vi "Master on Desktop — копия (2).vi"() -> ()   [LabVIEW 2021]
doc: "Demonstrates how to use Modbus functions to create a master communicating with a Modbus slave. It shows an interactive UI to allow users manually read and write the coils on the slave using TCP connection. Users can also change the timeout for reading operation if the network state is not good."
uses:
  subvis/Modbus API/Modbus API.lvclass/Modbus API.ctl
  subvis/Transmission Data Unit (ADU)/Transmission Data Unit/Transmission Data Unit.lvclass/Transmission Data Unit.ctl
  master/Data Access/Read Timeout/Set Read Timeout.vi
  subvis/Modbus API/Read Transmission Data Unit.vi
  subvis/Modbus API/Write Transmission Data Unit.vi
  subvis/Transmission Data Unit (ADU)/Transmission Data Unit/Data Access/timeouts/Write read operation timeout.vi
  master/Modbus Master.lvclass
  D:/my_projects/projects/Algorithms/Labview/21/Modbus_v2/subvis/Modbus API/Modbus API.lvclass
  master/Create Master Instance (TCP).vi
  subvis/Transmission Data Unit (ADU)/Transmission Data Unit/Transmission Data Unit.lvclass
panel:
  out "timer":u32(graph)
  in  "register values 2":u16[](array[numeric])
  out "register values":u16[](array[numeric])
  in  "Set Read Timeout":bool
  in  "Read Timeout (ms)":i32=5000
  in  "Read Count":u16=10
  in  "Stop":bool
  in  "Read":bool
  out "Coil Values Read":bool[](array[boolean])
  in  "Write":bool
  in  "Coil Values to Write":bool[](array[boolean])
  # "Overview: Demonstrates the use of the Modbus Master VIs to create a Modbus master and use the Modbus master to read and write coil values on a Modbus slave.\nRequirements: LabVIEW Datalogging and Supervisory Control Module\nInstructions:\n1. Ensure Slave On Desktop.vi is already running.\n2. Run the VI.\n3. Click Stop to stop the VI."
  # "Write Operation"
  # "Read Operation"
  # "Set Timeout For Read Operation"
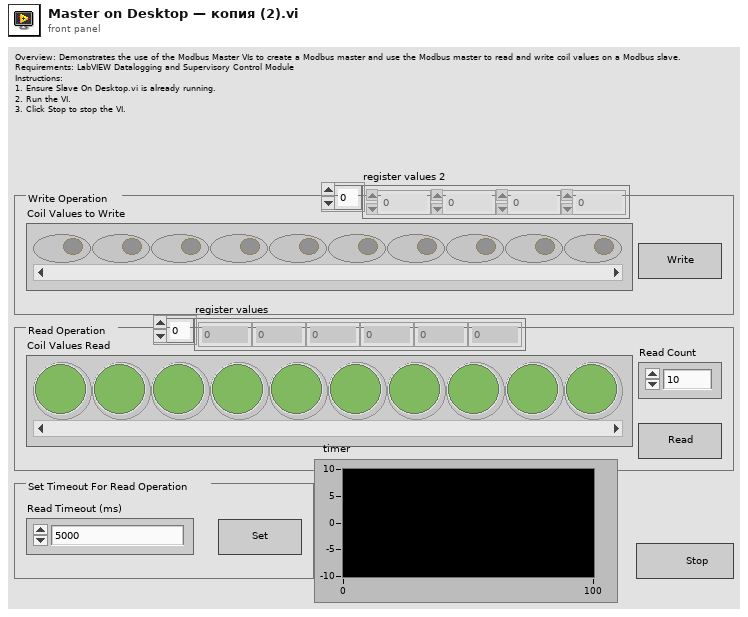
[diagram p1: front panel]
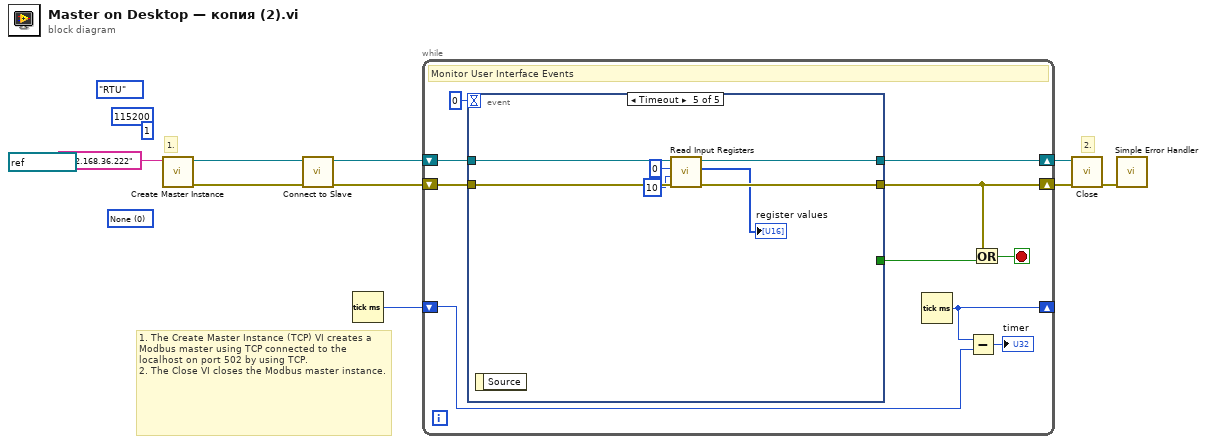
[diagram p0: block diagram]
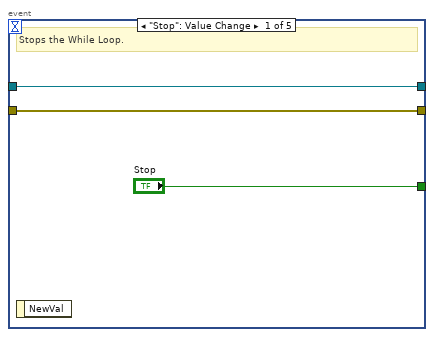
[diagram p2: hidden frame]
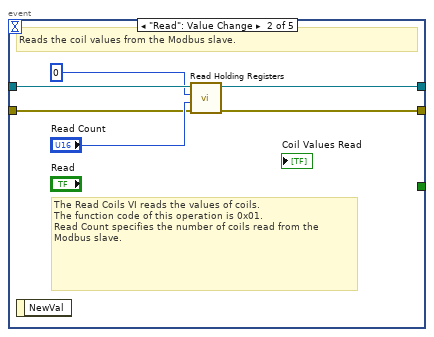
[diagram p3: hidden frame]
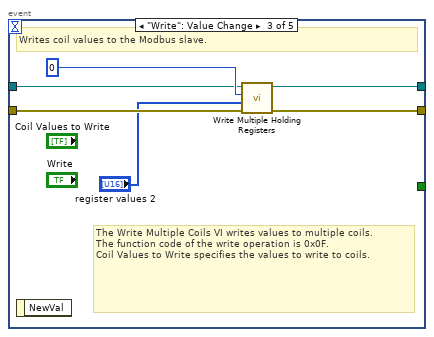
[diagram p4: hidden frame]
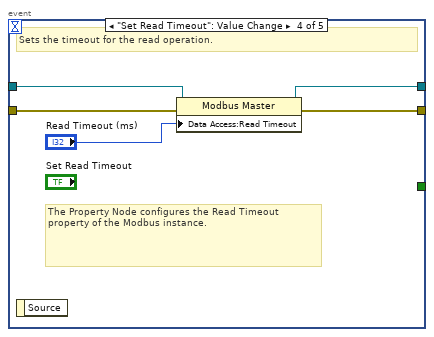
[diagram p5: hidden frame]
diagram:
  (unwired) refnum<visa-resource-name> "COM18" ("VISA resource name")
  (unwired) u16 0 items=["None", "Odd", "Even"] ("parity (Even)")
  (unwired) u32 115200 ("baud rate (9600)")
  (unwired) enum16{"RTU", "ASCII"}."RTU" ("serial type")
  (unwired) u8 1 ("unit ID")
  # "2."
  # "1."
  # "1. The Create Master Instance (TCP) VI creates a Modbus master using TCP connected to the localhost on port 502 by using TCP.\n2. The Close VI closes the Modbus master instance."
  n1 = call-poly "Create Master Instance.vi"("address"="192.168.36.222") -> ("error out"=w5:errorcluster, "TCP master instance"=w3:refnum<class "Modbus Master.lvclass">)  [unwired: 9 in]
  n2 = call-dynamic "Connect to Slave.vi"("error in (no error)"=w5, "Modbus master in"=w3) -> ("error out"=w4:errorcluster, "Modbus master out"=w6:refnum<class "Modbus Master.lvclass">)  [unwired: 8 in]
  n3 = Tick Count (ms)() -> (millisecond timer value=w2:u32)
  n4 = while {
    shift-right: [w18] -> w8
    shift-left: w6 -> [w19]
    shift-right: [w16] -> w9
    shift-left: w4 -> [w17]
    shift-right: [w11] -> _
    shift-left: w2 -> [w12]
    stop <- w14 stop-if-true
    # "Monitor User Interface Events"
    n5 = event shown="[4] Timeout" {
      selector: _ -> [_ _ _ _ _]
      dyn-events: _ -> [_ _ _ _ _]
      timeout: 0 -> [_ _ _ _ _]
      tunnel: ["Stop" _ _ _ _] -> w15
      tunnel: w19 -> [w21 w28 w33 w39 w46]
      tunnel: [w21 w27 w32 w37 w45] -> w18
      tunnel: w17 -> [w22 w24 w31 w38 w44]
      tunnel: [w22 w23 w30 w36 w43] -> w16
      event "Stop": Value Change {
        # "Stops the While Loop."
        n6 = event-data() -> ()  [unwired: 1 in, 1 out]
      }
      event "Read": Value Change {
        # "The Read Coils VI reads the values of coils.\nThe function code of this operation is 0x01.\nRead Count specifies the number of coils read from the Modbus slave."
        # "Reads the coil values from the Modbus slave."
        n7 = event-data() -> ()  [unwired: 1 in, 1 out]
        n8 = call-dynamic "Read Holding Registers.vi"("error in (no error)"=w24, "number of holding registers"="Read Count", "starting address"=u16 0, "Modbus master in"=w28) -> ("error out"=w23:errorcluster, "Modbus master out"=w27:refnum<class "Modbus Master.lvclass">)  [unwired: 5 in, 1 out]
      }
      event "Write": Value Change {
        # "The Write Multiple Coils VI writes values to multiple coils.\nThe function code of the write operation is 0x0F.\nCoil Values to Write specifies the values to write to coils."
        # "Writes coil values to the Modbus slave."
        n9 = event-data() -> ()  [unwired: 1 in, 1 out]
        n10 = call-dynamic "Write Multiple Holding Registers.vi"("error in (no error)"=w31, "holding register values"="register values 2", "starting address"=u16 0, "Modbus master in"=w33) -> ("error out"=w30:errorcluster, "Modbus master out"=w32:refnum<class "Modbus Master.lvclass">)  [unwired: 6 in]
      }
      event "Set Read Timeout": Value Change {
        # "The Property Node configures the Read Timeout property of the Modbus instance."
        # "Sets the timeout for the read operation."
        n11 = event-data() -> ()  [unwired: 1 in, 1 out]
        n12 = property class="Modbus Master"(reference=w39, error in=w38, "Data Access:Read Timeout"="Read Timeout (ms)") -> (reference out=w37:refnum<class "Modbus Master.lvclass">, error out=w36:errorcluster)
      }
      event Timeout {
        n13 = event-data() -> ()  [unwired: 1 in, 1 out]
        n14 = call-dynamic "Read Input Registers.vi"("error in (no error)"=w44, "number of input registers"=u16 10 ("number of holding registers"), "starting address"=u16 0, "Modbus master in"=w46) -> ("error out"=w43:errorcluster, "register values"=→"register values":u16[], "Modbus master out"=w45:refnum<class "Modbus Master.lvclass">)  [unwired: 5 in]
      }
    }
    n15 = Tick Count (ms)() -> (millisecond timer value=w11:u32)
    n16 = Subtract(x=w11, y=w12) -> (x-y=→"timer":u32)
    n17 = Or(x=w16, y=w15) -> (x .or. y?=w14:bool)
  }
  n18 = call-dynamic "Close.vi"("error in (no error)"=w9, "Modbus master in"=w8) -> ("error out"=w7:errorcluster)  [unwired: 9 in]
  n19 = call <vilib>:"Simple Error Handler.vi"("error in (no error)"=w7) -> ()  [unwired: 4 in, 5 out]
